vi "Initialize New.vi"(4 "Error In":errorcluster, 7 "Config Data_Text in":refnum<class "Config Data_Text.lvclass">) -> (0 "Error Out":errorcluster, 3 "Config Data_Text out":refnum<class "Config Data_Text.lvclass">)   [LabVIEW 2020, in "Config Data.lvlib" / "Config Data_Text.lvclass"]
uses:
  Config Data_Text.lvclass
  Config Data.lvclass
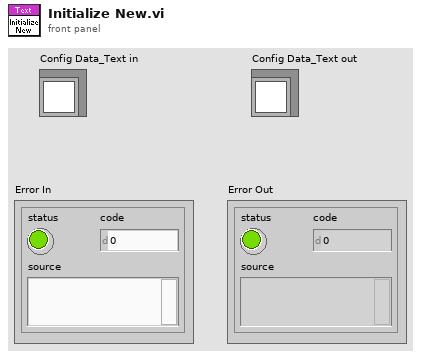
[diagram p1: front panel]
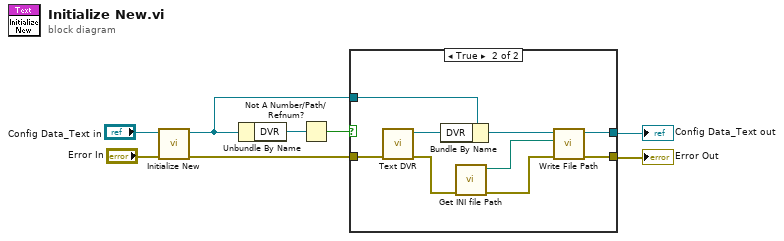
[diagram p0: block diagram]
diagram:
  n1 = call-parent "Initialize New.vi"("Error In"="Error In", "Config Data in"="Config Data_Text in") -> ("Error Out"=w3:errorcluster, "Config Data out"=w4:refnum<class "Config Data_Text.lvclass">)  [unwired: 4 in]
  n2 = Unbundle By Name(w4) -> ("DVR"=w6:refnum<data-value>)
  n3 = Not A Number/Path/Refnum?(number/path/refnum=w6) -> (NaN/Path/Refnum?=w5:bool)
  n4 = case shown="True" w5 {
    tunnel: w4 -> [w10 w19]
    tunnel: [w10 w11] -> w2
    tunnel: w3 -> [w9 w18]
    tunnel: [w9 w13] -> w1
    frame False {
    }
    frame True {
      n5 = call "Text DVR.vi"("Error In"=w18) -> ("Error Out"=w16:errorcluster, "DVR"=w17:refnum<data-value>)  [unwired: 5 in]
      n6 = Bundle By Name(cluster=w19, "DVR"=w17) -> (w12:refnum<class "Config Data_Text.lvclass">)
      n7 = call "Get INI file Path.vi"("error in (no error)"=w16) -> ("error out"=w14:errorcluster, "appended path"=w15:path)  [unwired: 5 in]
      n8 = call "Write File Path.vi"("Error In"=w14, "File Path"=w15, "Text In"=w12) -> ("Error Out"=w13:errorcluster, "Text Out"=w11:refnum<class "Config Data_Text.lvclass">)  [unwired: 3 in]
    }
  }
  "Error Out" <- w1
  "Config Data_Text out" <- w2
